vi "Create SignalWithAlarm.vi"(8 "error in (no error)":errorcluster, 10 "Low Limit":dbl=0.01, 11 "High Limit":dbl=0.99) -> (0 "error out":errorcluster, 3 "SignalWithAlarm out":refnum<class "SignalWithAlarm.lvclass">)   [LabVIEW 2016, in "SignalWithAlarm.lvclass"]
uses:
  SignalWithAlarm.lvclass
  SignalWithAlarm.lvclass/SignalWithAlarm.ctl
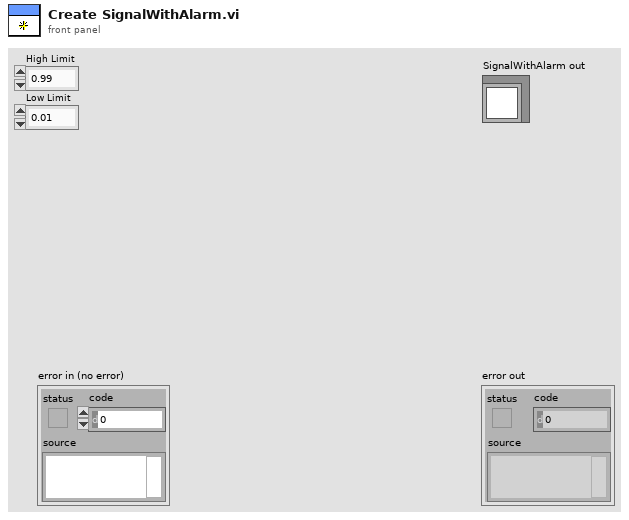
[diagram p1: front panel]
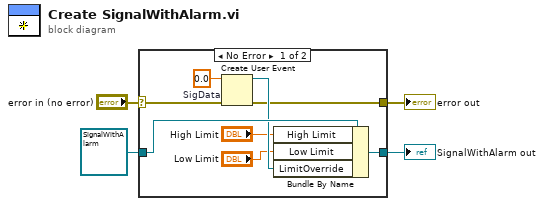
[diagram p0: block diagram]
diagram:
  n1 = case shown="No Error" "error in (no error)" {
    selector: "error in (no error)" -> [w5 w14]
    tunnel: [w6 w14] -> w3
    tunnel: [w11 w13] -> w1
    tunnel: refnum<class "SignalWithAlarm.lvclass"> refnum ("SignalWithAlarm in") -> [w12 w13]
    frame No Error {
      w9 = 0.0  # SigData
      n2 = Create User Event(user event datatype=w9, error in=w5) -> (user event=w10:refnum<user-event>, error out=w6:errorcluster)
      n3 = Bundle By Name(cluster=w12, "High Limit"="High Limit", "Low Limit"="Low Limit", "LimitOverride"=w10) -> (w11:refnum<class "SignalWithAlarm.lvclass">)
    }
    frame Error {
    }
  }
  "error out" <- w3
  "SignalWithAlarm out" <- w1
